vi "Get Reference Object Refnum.vi"(11 "LVClassLibrary in":refnum<vi>) -> (0 "error out":errorcluster, 2 "Found?":bool, 3 "LVObjectRefNum out":refnum<vi>)   [LabVIEW 2015, in "QControl Creation.lvclass"]
doc: "<b> </b> <b> </b>\n©2016 Q Software Innovations, LLC (QSI)\nwritten by Quentin Alldredge\nproduced in LabVIEW 2015\n\nsupport@qsoftwareinnovations.com\nwww.qsoftwareinnovations.com\n\nAll rights reserved.\n\nRedistribution and use in source and binary forms, with or without modification, are permitted provided that the following conditions are met:\n\n * Redistributions of source code must retain the above copyright notice, this list of conditions and the following disclaimer.\n * Redistributions in binary form must reproduce the above copyright notice, this list of conditions and the following disclaimer in the documentation and/or other materials provided with the distribution.\n * Neither the name of Q Software Innovations, LLC. nor the names of its contributors may be used to endorse or promote products derived from this software without specific prior written permission.\n\nTHIS SOFTWARE IS PROVIDED BY THE COPYRIGHT HOLDERS AND CONTRIBUTORS \"AS IS\" AND ANY EXPRESS OR IMPLIED WARRANTIES, INCLUDING, BUT NOT LIMITED TO, THE IMPLIED WARRANTIES OF MERCHANTABILITY AND FITNESS FOR A PARTICULAR PURPOSE ARE DISCLAIMED. IN NO EVENT SHALL THE COPYRIGHT OWNER OR CONTRIBUTORS BE LIABLE FOR ANY DIRECT, INDIRECT, INCIDENTAL, SPECIAL, EXEMPLARY, OR CONSEQUENTIAL DAMAGES (INCLUDING, BUT NOT LIMITED TO, PROCUREMENT OF SUBSTITUTE GOODS OR SERVICES; LOSS OF USE, DATA, OR PROFITS; OR BUSINESS INTERRUPTION) HOWEVER CAUSED AND ON ANY THEORY OF LIABILITY, WHETHER IN CONTRACT, STRICT LIABILITY, OR TORT (INCLUDING NEGLIGENCE OR OTHERWISE) ARISING IN ANY WAY OUT OF THE USE OF THIS SOFTWARE, EVEN IF ADVISED OF THE POSSIBILITY OF SUCH DAMAGE."
uses:
  QControl Creation.lvclass
  <vilib>/Utility/traverseref.llb/TRef TravTarget.ctl
  <vilib>/Utility/traverseref.llb/VI Scripting - Traverse.lvlib
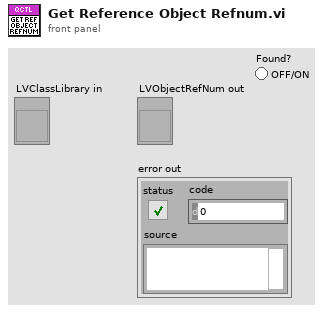
[diagram p1: front panel]
types:
  T1 = typedef "TRef TravTarget.ctl" = enum16{"FP", "BD", "Other"}
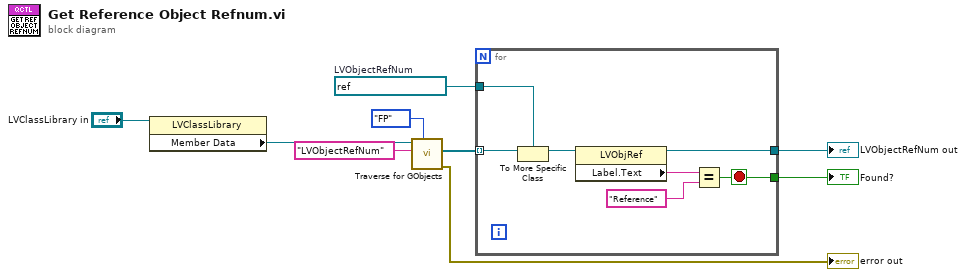
[diagram p0: block diagram]
diagram:
  w7 = refnum<vi> refnum  # LVObjectRefNum
  n1 = property class="LVClassLibrary"(reference="LVClassLibrary in") -> ("Member Data"=w4:refnum<vi>)  [unwired: 1 in, 2 out]
  n2 = call <vilib>:"Traverse for GObjects.vi"("Traverse Target"=TRef_TravTarget."FP", "Class Name"="LVObjectRefNum", "VI Refnum"=w4) -> ("error out"=→"error out":errorcluster, "References"=w5:refnum<vi>[])  [unwired: 5 in, 2 out]
  n3 = for {
    tunnel: w5 -> [w16] mode=indexing
    tunnel: w7 -> [w14]
    tunnel: [w11] -> w8
    tunnel: [w10] -> w1
    stop <- w10 stop-if-true
    n4 = To More Specific Class(target class=w14, reference=w16) -> (specific class reference=w15:refnum<vi>)  [unwired: 1 in, 1 out]
    n5 = property class="LVObjRef"(reference=w15) -> (reference out=w11:refnum<vi>, "Label.Text"=w13:string)  [unwired: 1 in, 1 out]
    n6 = Equal?(x=w13, y="Reference") -> (x = y?=w10:bool)
  }
  "LVObjectRefNum out" <- w8
  "Found?" <- w1
